vi "Alarm.vi"(5 "继承模式":string, 6 "提示":string, 7 "模式":enum16{"select", "insert", "update", "delete"}(ring), 8 "确认":bool, 9 "级别":string, 10 "类型":string, 11 "消息名":string) -> (2 "data":string[][](array[string]))   [LabVIEW 2012]
uses:
  <vilib>/addons/database/_DB Variant To Data/Database Variant To Data.xnode
panel:
  out "SQL query":string
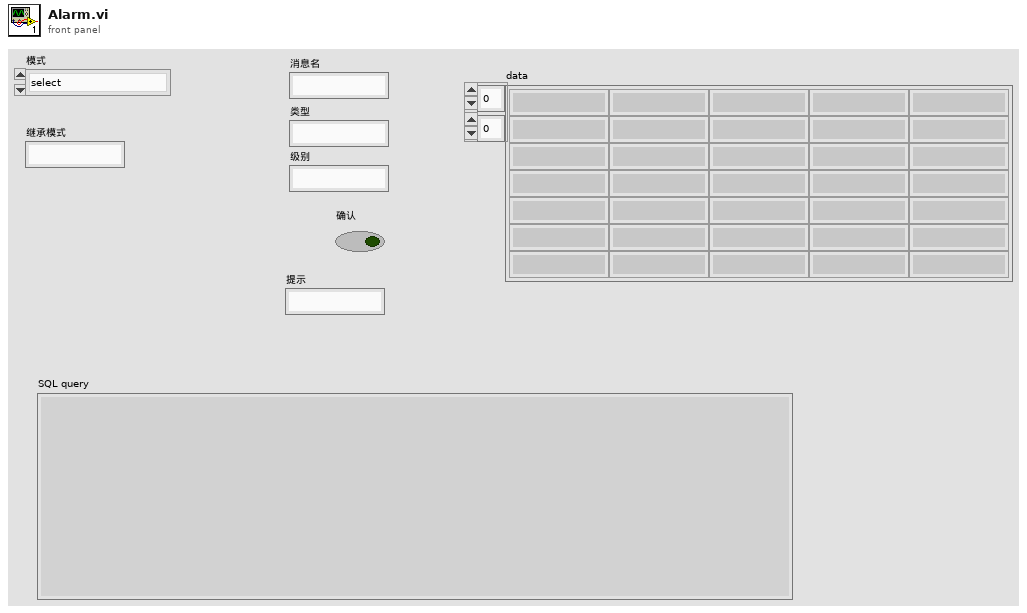
[diagram p1: front panel]
types:
  T1 = cluster{"type":string, "level":string, "datatime":string, "check":string, "tips":string}
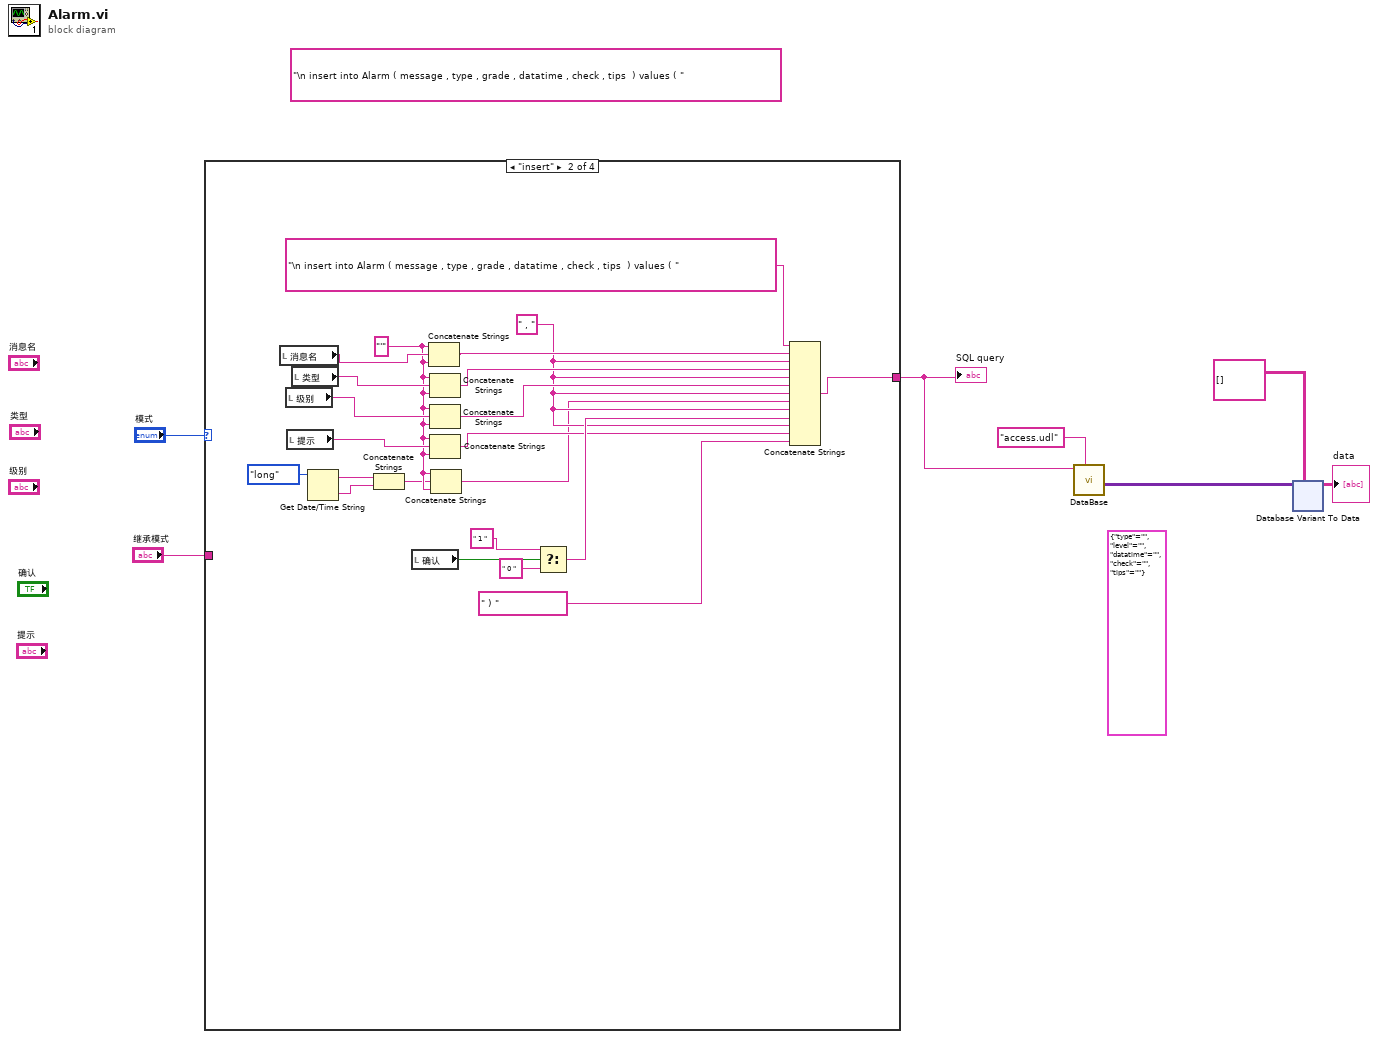
[diagram p0: block diagram]
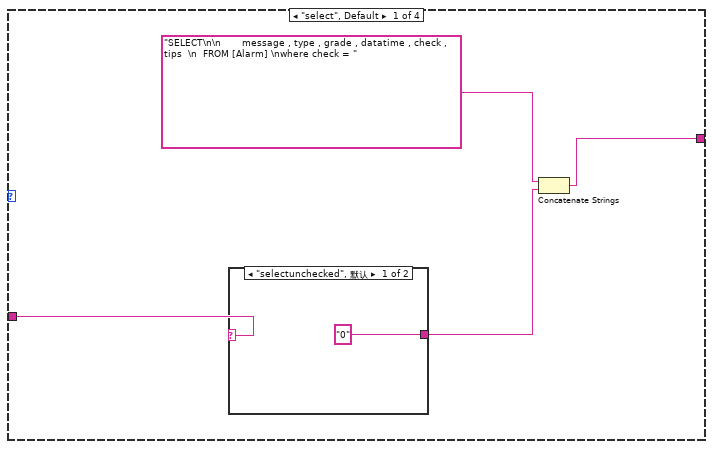
[diagram p2: hidden frame]
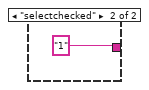
[diagram p3: hidden frame]
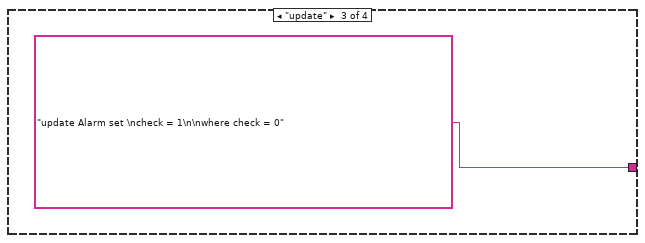
[diagram p4: hidden frame]
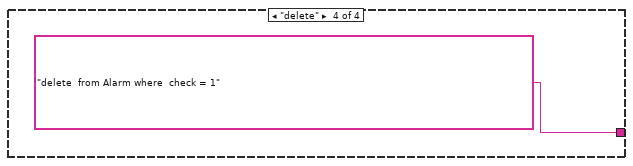
[diagram p5: hidden frame]
diagram:
  (unwired) T1 {"type"="", "level"="", "datatime"="", "check"="", "tips"=""}
  (unwired) "\n insert into Alarm ( message , type , grade , datatime , check , tips  ) values ( " ("SQL query")
  n1 = case shown="\"insert\"" "模式" {
    tunnel: [w11 w21 "update Alarm set \ncheck = 1\n\nwhere check = 0" ("SQL query") "delete  from Alarm where  check = 1" ("SQL query")] -> w3
    tunnel: "继承模式" -> [w9 _ _ _]
    frame "select", Default {
      n2 = case shown="\"selectunchecked\", 默认" w9 {
        tunnel: ["0" ("udl名称") "1" ("udl名称")] -> w8
        frame "selectunchecked", Default {
        }
        frame "selectchecked" {
        }
      }
      n3 = Concatenate Strings("SELECT\n\n       message , type , grade , datatime , check , tips  \n  FROM [Alarm] \nwhere check = " ("SQL query"), w8) -> (w11:string)
    }
    frame "insert" {
      w16 = "'"
      w19 = " , "
      n4 = local read "消息名"() -> (w33:string)
      n5 = local read "级别"() -> (w29:string)
      n6 = local read "提示"() -> (w20:string)
      n7 = local read "类型"() -> (w31:string)
      n8 = Get Date/Time String ("获取日期/时间字符串")(date format (0)=enum16{"short", "long", "abbreviated"}."long" ("日期格式(0)")) -> (date string=w25:string, time string=w24:string)  [unwired: 2 in]
      n9 = Concatenate Strings(w25, w24) -> (w14:string)
      n10 = local read "确认"() -> (w35:bool)
      n11 = Concatenate Strings(w16, w33, w16) -> (w32:string)
      n12 = Concatenate Strings(w16, w31, w16) -> (w30:string)
      n13 = Concatenate Strings(w16, w29, w16) -> (w28:string)
      n14 = Concatenate Strings(w16, w20, w16) -> (w17:string)
      n15 = Concatenate Strings(w16, w14, w16) -> (w15:string)
      n16 = Select(t=" 1 ", s=w35, f=" 0 ") -> (s? t:f=w34:string)
      n17 = Concatenate Strings("\n insert into Alarm ( message , type , grade , datatime , check , tips  ) values ( " ("SQL query"), w32, w19, w30, w19, w28, w19, w15, w19, w34, w19, w17, " ) " ("SQL query")) -> (w21:string)
    }
    frame "update" {
    }
    frame "delete" {
    }
  }
  "SQL query" <- w3
  n18 = call "DataBase.vi"("udl名称"="access.udl", "SQL query"=w3) -> ("recordset data"=w5:variant[][])  [unwired: 9 in]
  n19 = xnode ("Database Variant To Data")("database variant"=w5, "type"=string[][] [] ("添加的数组")) -> ("data"=→"data":string[][])  [unwired: 1 in, 1 out]
